vi "bPM.vi"() -> ()   [LabVIEW 2015]
uses:
  <vilib>/Analysis/3filter.llb/Filter Passband Type.ctl
  <vilib>/ptbypt/NI_PtbyPt.lvlib
  <vilib>/Analysis/NI_AALBase.lvlib
panel:
  out "Waveform Chart":dbl(graph)
  out "BPM":dbl
  in  "inatilize":bool
  out "filter Chart":dbl(graph)
  in  "stop":bool
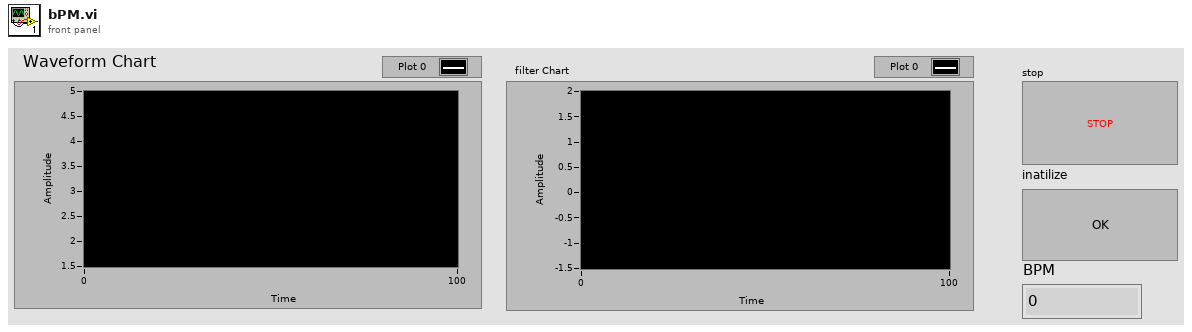
[diagram p1: front panel]
types:
  T1 = typedef "NI_AALBase.lvlib/Filter Passband Type.ctl" = enum32{"Lowpass", "Highpass", "Bandpass", "Bandstop"}
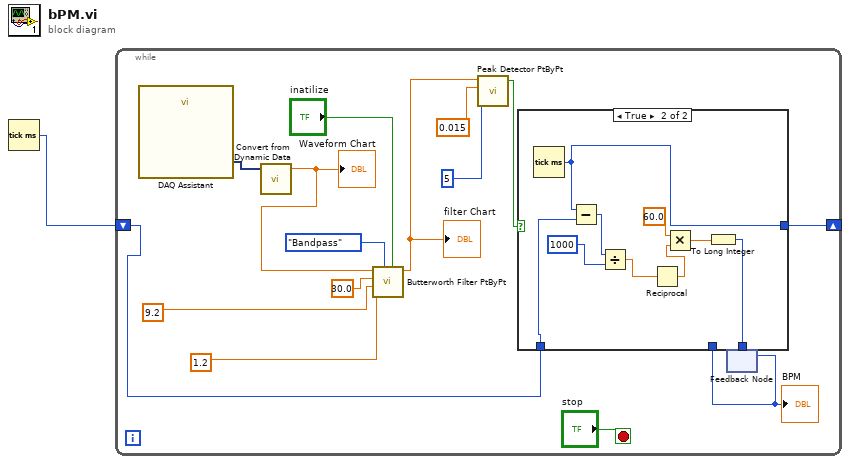
[diagram p0: block diagram]
diagram:
  n1 = Tick Count (ms)() -> (millisecond timer value=w1:u32)
  n2 = while {
    shift-right: [w8] -> _
    shift-left: w1 -> [w9]
    stop <- "stop" stop-if-true
    n3 = call "DAQ Assistant"() -> ("data"=w4:dynamicdata)  [unwired: 16 in, 3 out]
    n4 = call "Convert from Dynamic Data"("Dynamic Data Type"=w4) -> ("Scalar"=w5:dbl)  [unwired: 3 in]
    "Waveform Chart" <- w5
    n5 = call <vilib>:"Butterworth Filter PtByPt.vi"("initialize"="inatilize", "filter type"=Filter_Passband_Type."Bandpass", "low cutoff freq: fl"=1.2, "high cutoff freq: fh"=9.2, "sampling freq: fs"=30.0, "x"=w5) -> ("Filtered x"=w13:dbl)  [unwired: 3 in, 1 out]
    "filter Chart" <- w13
    n6 = call <vilib>:"Peak Detector PtByPt.vi"("x"=w13, "threshold peak"=0.015, "width"=5) -> ("peak"=w10:bool)  [unwired: 2 in, 2 out]
    n7 = feedback #1() -> (w6:i32)  [unwired: 1 in]
    "BPM" <- w6
    n8 = case shown="True" w10 {
      tunnel: w9 -> [w19 w28]
      tunnel: [w19 w25] -> w8
      tunnel: [w18 w24] -> w7
      tunnel: w6 -> [w18 _]
      frame False {
      }
      frame True {
        n9 = Tick Count (ms)() -> (millisecond timer value=w25:u32)
        n10 = Subtract(x=w25, y=w28) -> (x-y=w22:u32)
        n11 = Divide(x=w22, y=u32 1000) -> (x/y=w21:dbl)
        n12 = Reciprocal(x=w21) -> (1/x=w20:dbl)
        n13 = Multiply(x=60.0, y=w20) -> (x*y=w26:dbl)
        n14 = To Long Integer(number=w26) -> (32bit integer=w24:i32)
      }
    }
    n15 = feedback-in #1(w7) -> ()
  }
